vi "DC Voltage Source.vi"() -> ()   [LabVIEW 2015]
panel:
  out "error out":errorcluster
  in  "Stop Button":bool
  in  "Voltage":dbl format="%#.3g"
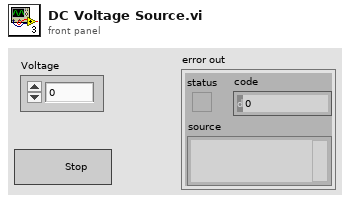
[diagram p1: front panel]
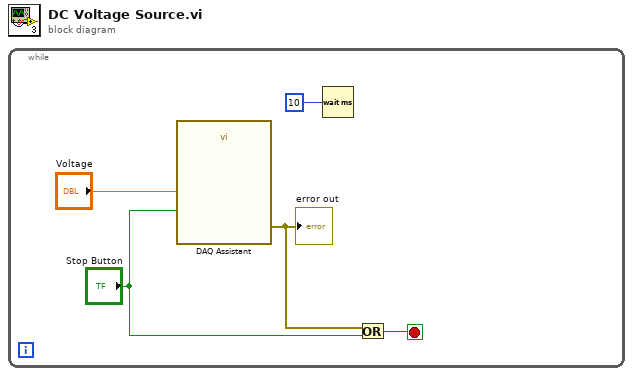
[diagram p0: block diagram]
diagram:
  n1 = while {
    stop <- w2 stop-if-true
    n2 = call "DAQ Assistant"("data"="Voltage", "stop (T)"="Stop Button") -> ("error out"=w1:errorcluster)  [unwired: 16 in, 1 out]
    "error out" <- w1
    n3 = Wait (ms)(milliseconds to wait=u32 10 ("millisecond timer value")) -> ()  [unwired: 1 out]
    n4 = Or(x=w1, y="Stop Button") -> (x .or. y?=w2:bool)
  }
